vi "cam_initialize.vi"(8 "error in (no error)":errorcluster, 10 "Robot ID":string="Picture", 11 "SceneGraphDisplay in":refnum<vi>) -> (0 "error out":errorcluster, 1 "camera image":T2, 2 "camera ref":refnum<k20>, 3 "SceneGraphDisplay out":refnum<vi>, 4 "camera values":T1)   [LabVIEW 2018]
uses:
  <vilib>/vision/Image Controls.llb/IMAQ Image.ctl
  <vilib>/robotics/Simulator/Interface/Simulator References/Get Sensor Reference.vi
  <vilib>/robotics/Simulator/NI_Robotics_Simulator.lvlib
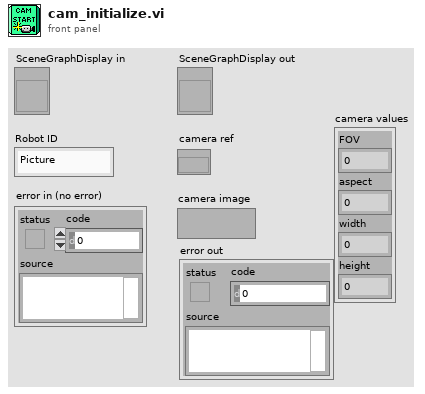
[diagram p1: front panel]
types:
  T1 = cluster{"FOV":dbl, "aspect":dbl, "width":dbl, "height":dbl}
  T2 = typedef "IMAQ Image.ctl" = refnum<image>
  T3 = typedef "Image Type" = u32
  T4 = cluster{"Robot ID":string, "sensor/actuator ID":string}
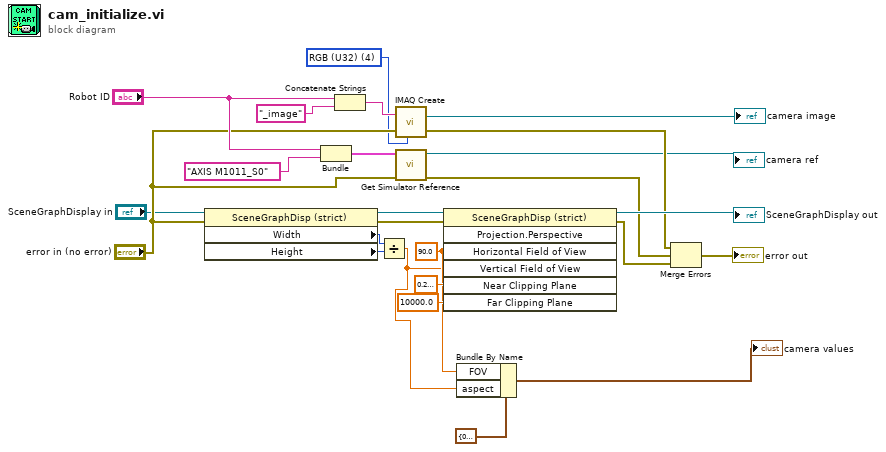
[diagram p0: block diagram]
diagram:
  w5 = T3 4 items=["Grayscale (U8)", "Grayscale (I16)", "Grayscale (SGL)", "Complex (CSG)", "RGB (U32)", "HSL (U32)", "RGB (U64)", "Grayscale (U16)"] ("Image Type")
  w3 = sgl 90.0 ("Field of View")
  n1 = property on="Property Node" class="SceneGraphDisp (strict)"(reference="SceneGraphDisplay in", error in="error in (no error)") -> (reference out=w16:refnum<vi>, error out=w17:errorcluster, "Width"=w11:u32, "Height"=w12:u32)
  n2 = Bundle("Robot ID"="Robot ID", "sensor/actuator ID"="AXIS M1011_S0") -> (w19:T4)  [unwired: 1 in]
  n3 = Concatenate Strings("Robot ID", "_image" ("Image Name")) -> (w21:string)
  n4 = Divide(x=w11, y=w12) -> (x/y=w2:dbl)
  n5 = call "IMAQ Create"("Image Name"=w21, "Image Type"=w5, "error in (no error)"="error in (no error)") -> ("New Image"=→"camera image":T2, "error out"=w10:errorcluster)  [unwired: 1 in, 1 out]
  n6 = call-poly <vilib>:"Get Simulator Reference.vi"("error in (no error)"="error in (no error)", "device ID"=w19) -> ("error out"=w9:errorcluster, "sensor ref"=→"camera ref":refnum<k20>)  [unwired: 8 in]
  n7 = invoke on="Invoke Node" class="SceneGraphDisp (strict)" method="Projection.Perspective"(reference=w16, error in=w17, "Horizontal Field of View"=w3, "Vertical Field of View"=w2, "Near Clipping Plane"=sgl 0.2, "Far Clipping Plane"=sgl 10000.0) -> (reference out=→"SceneGraphDisplay out":refnum<vi>, error out=w8:errorcluster)  [unwired: 1 in, 5 out]
  n8 = Bundle By Name(cluster=T1 {"FOV"=0.0, "aspect"=0.0, "width"=0.0, "height"=0.0}, "FOV"=w3, "aspect"=w2) -> (→"camera values":T1)
  n9 = Merge Errors(w10, w9, w8) -> (→"error out":errorcluster)
